vi "Update GraphChart LegendSize.vi"(0 "GraphChart Reference":refnum<vi>, 1 "# Plots":i32, 3 "error in (no error)":errorcluster, 4 "Display Type":enum16{"Chart", "Graph"}(ring)) -> (5 "GraphChart Reference out":refnum<vi>, 6 "error out":errorcluster)   [LabVIEW 2015]
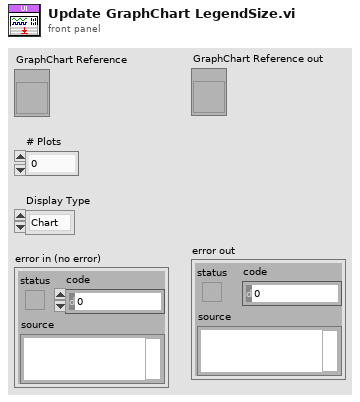
[diagram p1: front panel]
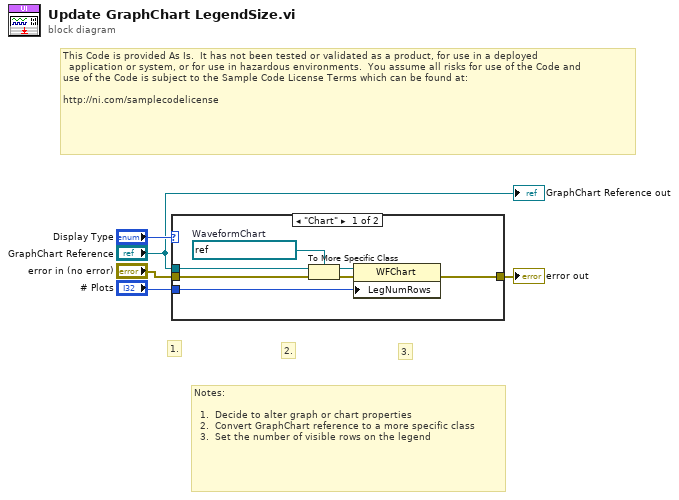
[diagram p0: block diagram]
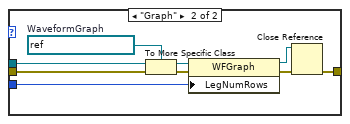
[diagram p2: hidden frame]
diagram:
  # "This Code is provided As Is.  It has not been tested or validated as a product, for use in a deployed\n  application or system, or for use in hazardous environments.  You assume all risks for use of the Code and   \nuse of the Code is subject to the Sample Code License Terms which can be found at: \n\nhttp://ni.com/samplecodelicense"
  # "Notes:  \n\n  1.  Decide to alter graph or chart properties  \n  2.  Convert GraphChart reference to a more specific class  \n  3.  Set the number of visible rows on the legend"
  # "3."
  # "2."
  # "1."
  n1 = case shown="\"Chart\"" "Display Type" {
    tunnel: [w6 w16] -> w2
    tunnel: "error in (no error)" -> [w10 w15]
    tunnel: "# Plots" -> [w8 w14]
    tunnel: "GraphChart Reference" -> [w7 w13]
    frame "Chart" {
      w12 = refnum<vi> refnum  # WaveformChart
      n2 = To More Specific Class(target class=w12, reference=w7, error in=w10) -> (specific class reference=w11:refnum<vi>, error out=w9:errorcluster)
      n3 = property class="WFChart"(reference=w11, error in=w9, "LegNumRows"=w8) -> (error out=w6:errorcluster)  [unwired: 1 out]
    }
    frame "Graph" {
      w21 = refnum<vi> refnum  # WaveformGraph
      n4 = To More Specific Class(target class=w21, reference=w13, error in=w15) -> (specific class reference=w20:refnum<vi>, error out=w19:errorcluster)
      n5 = property class="WFGraph"(reference=w20, error in=w19, "LegNumRows"=w14) -> (reference out=w18:refnum<vi>, error out=w17:errorcluster)
      n6 = Close Reference(reference=w18, error in (no error)=w17) -> (error out=w16:errorcluster)
    }
  }
  "error out" <- w2
  "GraphChart Reference out" <- "GraphChart Reference"
